vi "excursion.vi"() -> ()   [LabVIEW 2020]
uses:
  From/System_conf.ctl
panel:
  in  "Sensor":T1
  in  "excursion":T2
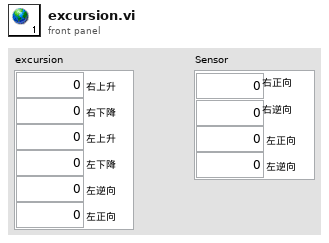
[diagram p1: front panel]
types:
  T1 = cluster{"右正向":dbl, "右逆向":dbl, "左正向":dbl, "左逆向":dbl}
  T2 = typedef "System_conf.ctl" = cluster{"右上升":dbl, "右下降":dbl, "左上升":dbl, "左下降":dbl, "左逆向":dbl, "左正向":dbl}
diagram:
